vi "TCP Server 单向通信.vi"() -> ()   [LabVIEW 2015]
uses:
  <vilib>/measure/NI_MABase.lvlib
panel:
  in  "local port":u16
  in  "signal type":T1(ring)
  in  "stop":bool
  out "Waveform Graph":waveform(dbl)(graph)
  in  "amplitude":dbl=1.0 format="%0.2p"
  in  "frequency":dbl=10.0 format="%0.2p"
  out "remote port":u16
  out "remote address":string
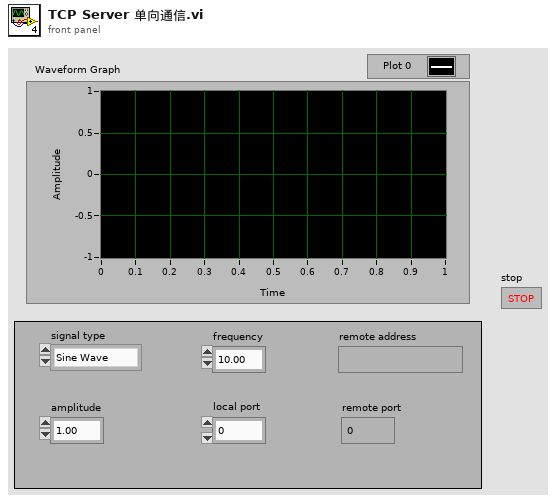
[diagram p1: front panel]
types:
  T1 = enum16{"Sine Wave", "Triangle Wave", "Square Wave", "Sawtooth Wave"}
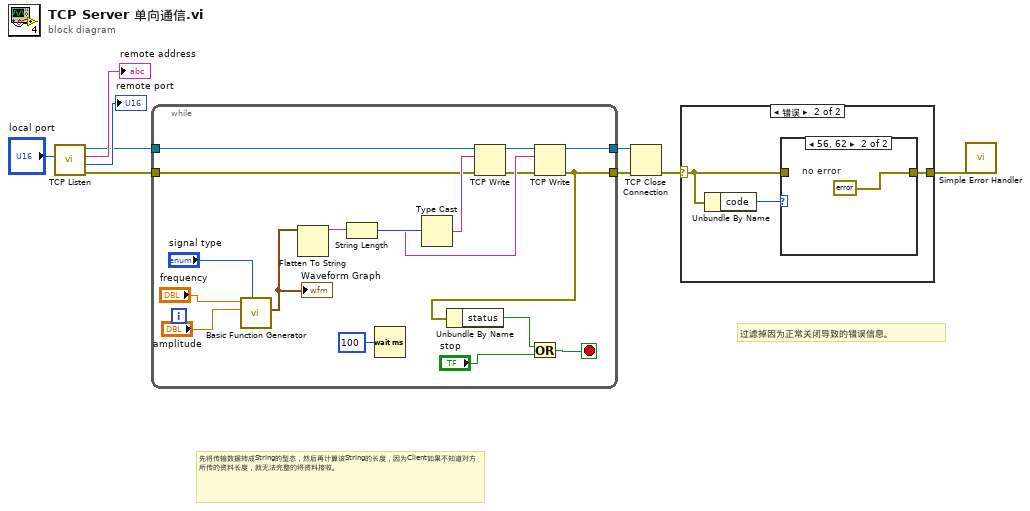
[diagram p0: block diagram]
diagram:
  # "过滤掉因为正常关闭导致的错误信息。"
  # "先将传输数据转成String的型态，然后再计算该String的长度，因为Client如果不知道对方所传的资料长度，就无法完整的将资料接收。"
  n1 = call <vilib>:"TCP Listen.vi"("port"="local port") -> ("error out"=w6:errorcluster, "remote port"=→"remote port":u16, "remote address"=→"remote address":string, "connection ID"=w7:refnum<k5>)  [unwired: 6 in, 1 out]
  n2 = while {
    tunnel: w7 -> [w22]
    tunnel: w6 -> [w14]
    tunnel: [w15] -> w5
    tunnel: [w21] -> w4
    stop <- w12 stop-if-true
    n3 = call <vilib>:"Basic Function Generator.vi"("signal type"="signal type", "amplitude"="amplitude", "frequency"="frequency") -> ("signal out"=w19:waveform(dbl))  [unwired: 6 in, 2 out]
    "Waveform Graph" <- w19
    n4 = Flatten To String(anything=w19) -> (data string=w17:string)  [unwired: 3 in, 2 out]
    n5 = String Length(string=w17) -> (length=w25:i32)
    n6 = Wait (ms)(milliseconds to wait=u32 100) -> ()  [unwired: 1 out]
    n7 = Type Cast(x=w25) -> (*(type *) &x=w24:string)  [unwired: 1 in]
    n8 = TCP Write(connection ID=w22, data in=w24, error in (no error)=w14) -> (connection ID out=w23:refnum<k5>, error out=w13:errorcluster)  [unwired: 1 in, 1 out]
    n9 = TCP Write(connection ID=w23, data in=w17, error in (no error)=w13) -> (connection ID out=w21:refnum<k5>, error out=w15:errorcluster)  [unwired: 1 in, 1 out]
    n10 = Unbundle By Name(w15) -> ("status"=w10:bool)
    n11 = Or(x=w10, y="stop") -> (x .or. y?=w12:bool)
  }
  n12 = TCP Close Connection(connection ID=w4, error in (no error)=w5) -> (error out=w2:errorcluster)  [unwired: 1 in, 1 out]
  n13 = case shown="错误" w2 {
    selector: w2 -> [w27 w29]
    tunnel: [w27 w30] -> w1
    frame No Error {
    }
    frame Error {
      n14 = Unbundle By Name(w29) -> ("code"=w28:i32)
      n15 = case shown="56, 62" w28 {
        tunnel: [w31 w32] -> w30
        tunnel: w29 -> [w31 _]
        frame Default {
        }
        frame 56, 62 {
          w32 = errorcluster {"status"=FALSE, "code"=0, "source"=""}  # no error
        }
      }
    }
  }
  n16 = call <vilib>:"Simple Error Handler.vi"("error in (no error)"=w1) -> ()  [unwired: 4 in, 5 out]
